vi "Get Channel Count.vi"(8 "error in (no error)":errorcluster, 11 "Transfer Configuration in":refnum<class "Configuration.Transfer.lvclass">) -> (0 "error out":errorcluster, 2 "channel count":i32, 3 "Transfer Configuration out":refnum<class "Configuration.Transfer.lvclass">)   [LabVIEW 2016, in "Configuration.Transfer.lvclass"]
uses:
  Configuration.Transfer.lvclass
  Configuration.Transfer.lvclass/Configuration.Transfer.ctl
  Configuration.Channel/Configuration.Channel.lvclass
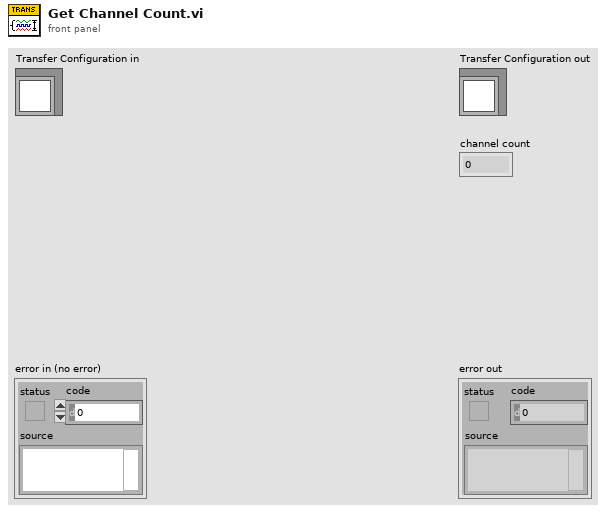
[diagram p1: front panel]
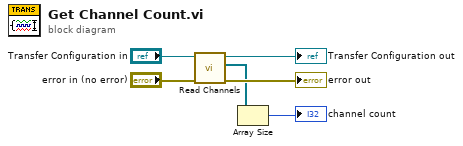
[diagram p0: block diagram]
diagram:
  n1 = call "Read Channels.vi"("error in (no error)"="error in (no error)", "Configuration.Transfer in"="Transfer Configuration in") -> ("error out"=→"error out":errorcluster, "Channels"=w2:refnum<class "Configuration.Channel.lvclass">[], "Configuration.Transfer out"=→"Transfer Configuration out":refnum<class "Configuration.Transfer.lvclass">)  [unwired: 7 in]
  n2 = Array Size(array=w2) -> (size(s)=→"channel count":i32)
